vi "ProcessAlways.vi"(0 "StateIn":T2 {"ILoad" format="%_6g"; "Fault Registers" format="%016x"; "VLoad" format="%_6g"; "VDCLink" format="%_6g"; "Detected Frequency" format="%1_6g"}, 1 "Interfaces":T5, 11 "error in":errorcluster) -> (4 "StateOut":T2 {"ILoad" format="%_6g"; "Fault Registers" format="%016x"; "VLoad" format="%_6g"; "VDCLink" format="%_6g"; "Detected Frequency" format="%1_6g"}, 8 "method":T1, 10 "params":refnum<class "JSON Null.lvclass">, 15 "error out":errorcluster)   [LabVIEW 2017, in "AppStateMachine runtime.lvclass"]
uses:
  AppStateMachine runtime.lvclass
  Interfaces.ctl
  <vilib>/NI/NI JSONRPC Server Framework/Classes/Server/JSONRPC Server.lvclass
  <instrlib>/_niInstr/Instruction Framework/v1/Host/Instruction Target/niInstr Instruction Target v1 Host.lvclass
  <instrlib>/_niInstr/Instruction Framework/v1/Host/Instruction Framework Context/niInstr Instruction Framework Context v1 Host.lvclass
  FPGA/FPGAtypedef.ctl
  <vilib>/NI/PowerElectronicsControl/ThreePhasePLL/Interface/InterfaceRef.ctl
  <vilib>/NI/PowerElectronicsControl/ActiveFrontEnd/AFE_Interface/InterfaceRef.ctl
  <vilib>/NI/PowerElectronicsControl/Buck-Boost/RealTime/Interface.ctl
  State.ctl
  StateId.ctl
  LED_Color.ctl
  Support/methods.ctl
  <vilib>/NI/JSON Support for LabVIEW/JSON Data Classes/JSON Datatype/JSON Null.lvclass
  <vilib>/NI/NI JSONRPC Server Framework/Classes/Request/Request.lvclass/Request.ctl
  <vilib>/NI/NI JSONRPC Server Framework/Classes/Request/Read method.vi
  <vilib>/NI/NI JSONRPC Server Framework/Classes/Request/Read params.vi
  <vilib>/NI/JSON Support for LabVIEW/JSON Data Classes/JSON Object/JSON Object.lvclass
  C:/Program Files (x86)/National Instruments/LabVIEW 2017/vi.lib/NI/JSON Support for LabVIEW/JSON Data Classes/JSON Datatype/JSON Null.lvclass
  <vilib>/NI/JSON Support for LabVIEW/JSON Data Classes/JSON String/JSON String.lvclass
  <vilib>/NI/JSON Support for LabVIEW/JSON Data Classes/JSON Array/JSON Array.lvclass
  <vilib>/NI/NI JSONRPC Server Framework/Classes/Server/Add Response (Method Not Found from Request).vi
  <vilib>/NI/NI JSONRPC Server Framework/Classes/Server/Add Response (Result from Request).vi
  <vilib>/NI/JSON Support for LabVIEW/JSON Data Classes/JSON String/New JSON String.vi
  <vilib>/NI/JSON Support for LabVIEW/JSON Data Classes/JSON Array/New JSON Array (String).vi
  <vilib>/NI/JSON Support for LabVIEW/JSON Data Classes/JSON Array/New JSON Array (JSON Data).vi
  <vilib>/Utility/error.llb/Error Cluster From Error Code.vi
  <vilib>/rvi/errors/niLvFpgaAdjustHostInterfaceError.vi
  <vilib>/NI/JSON Support for LabVIEW/JSON Data Classes/JSON Object/New JSON Object (Empty).vi
  <vilib>/rvi/interface/nirviReadWriteControl/nirviReadWriteControl.xnode
  <vilib>/NI/NI JSONRPC Server Framework/Classes/params/params.lvclass
  <vilib>/rvi/interface/Simulation/niFpgaSimulationCallBeginRW.vi
  <vilib>/NI/PowerElectronicsControl/ThreePhasePLL/Interface/ThreePhasePLLInterface.lvlib
  <vilib>/NI/JSON Support for LabVIEW/JSON Data Classes/JSON Helper/JSON Helper.lvclass
  NiFpgaLv.dll
  <vilib>/NI/NI JSONRPC Server Framework/Classes/Request/Request.lvclass
  C:/Program Files (x86)/National Instruments/LabVIEW 2017/vi.lib/NI/JSON Support for LabVIEW/JSON Data Classes/JSON Basic Type/JSON Literal.lvclass
  C:/Program Files (x86)/National Instruments/LabVIEW 2017/vi.lib/NI/JSON Support for LabVIEW/JSON Data Classes/JSON Structured Type/JSON Structure.lvclass
  <vilib>/NI/PowerElectronicsControl/Buck-Boost/RealTime/BuckBoostInterface.lvlib
  <vilib>/NI/PowerElectronicsControl/ActiveFrontEnd/AFE_Interface/AFE_interface.lvlib
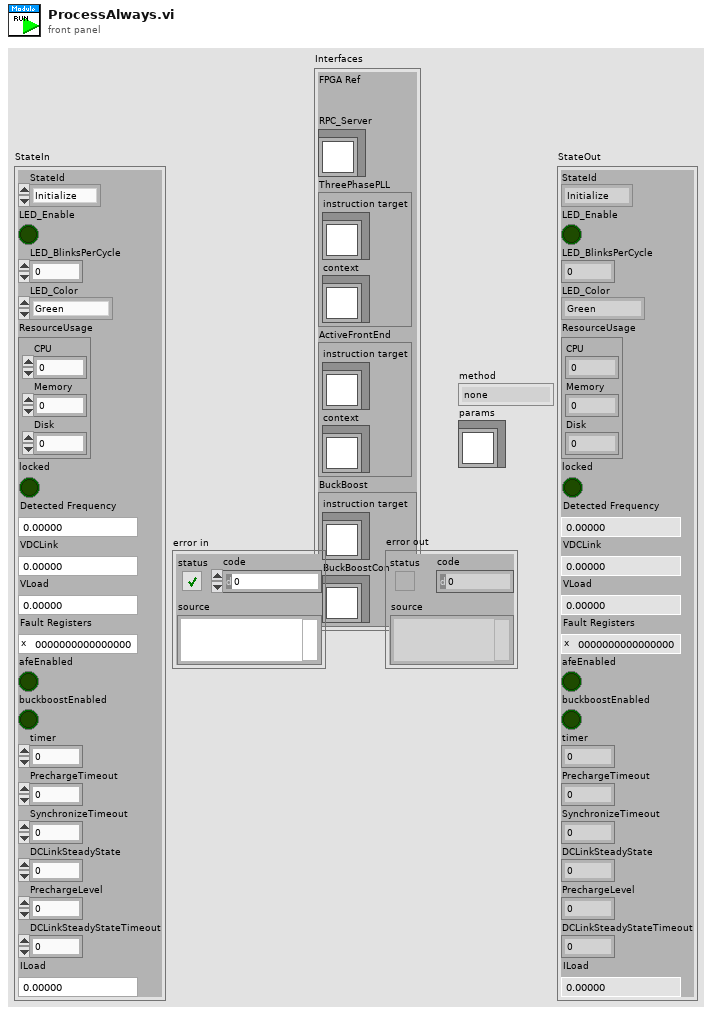
[diagram p1: front panel]
types:
  T1 = typedef "AppStateMachine runtime.lvclass/methods.ctl" = enum16{"none", "echo", "GetResourceUsage", "CheckConnection", "CurrentState", "GoToSafeState", "ClearSafeState", "AvailableLogs", "ForceLogTrigger", "GoToTuneAFE", "GoToTunePLL", "GoToTuneBuckBoost", "TurnOnSystem", "TurnOffSystem", "PrechargeSystem", "SetPLL_Tune", "SetBuckBoostSetpoint", "SetAFE_tune", "SetBuckBoostTune", "CompleteTuning", "PllSettings", "AfeSettings", "BuckBoostSettings", "enableAfe", "disableAfe", "enableBuckBoost", "disableBuckBoost"}
  T2 = typedef "AppStateMachine runtime.lvclass/State.ctl" = cluster{"StateId":T3, "LED_Enable":bool, "LED_BlinksPerCycle":i32, "LED_Color":T4, "ResourceUsage":cluster{"CPU":dbl, "Memory":dbl, "Disk":dbl}, "locked":bool, "Detected Frequency":dbl, "VDCLink":dbl, "VLoad":dbl, "Fault Registers":u64, "afeEnabled":bool, "buckboostEnabled":bool, "timer":u32, "PrechargeTimeout":u32, "SynchronizeTimeout":u32, "DCLinkSteadyState":dbl, "PrechargeLevel":dbl, "DCLinkSteadyStateTimeout":u32, "ILoad":dbl}
  T3 = typedef "AppStateMachine runtime.lvclass/StateId.ctl" = enum16{"Initialize", "Idle", "TunePLL", "TuneAFE", "TuneBuckBoost", "Precharge", "Synchronize", "Ready", "EnableAFE", "EnableBuckBoost", "Powered", "SafeState", "UnrecoverableSafeState"}
  T4 = typedef "AppStateMachine runtime.lvclass/LED_Color.ctl" = enum16{"Green", "Yellow"}
  T5 = typedef "AppStateMachine runtime.lvclass/Interfaces.ctl" = cluster{"FPGA Ref":T6, "RPC_Server":refnum<class "JSONRPC Server.lvclass">, "ThreePhasePLL":T7, "ActiveFrontEnd":T8, "BuckBoost":T9}
  T6 = typedef "AppStateMachine runtime.lvclass/FPGAtypedef.ctl" = refnum<k20>
  T7 = typedef "ThreePhasePLLInterface.lvlib/InterfaceRef.ctl" = cluster{"instruction target":refnum<class "niInstr Instruction Target v1 Host.lvclass">, "context":refnum<class "niInstr Instruction Framework Context v1 Host.lvclass">}
  T8 = typedef "AFE_interface.lvlib/InterfaceRef.ctl" = cluster{"instruction target":refnum<class "niInstr Instruction Target v1 Host.lvclass">, "context":refnum<class "niInstr Instruction Framework Context v1 Host.lvclass">}
  T9 = typedef "BuckBoostInterface.lvlib/Interface.ctl" = cluster{"instruction target":refnum<class "niInstr Instruction Target v1 Host.lvclass">, "BuckBoostContext":refnum<class "niInstr Instruction Framework Context v1 Host.lvclass">}
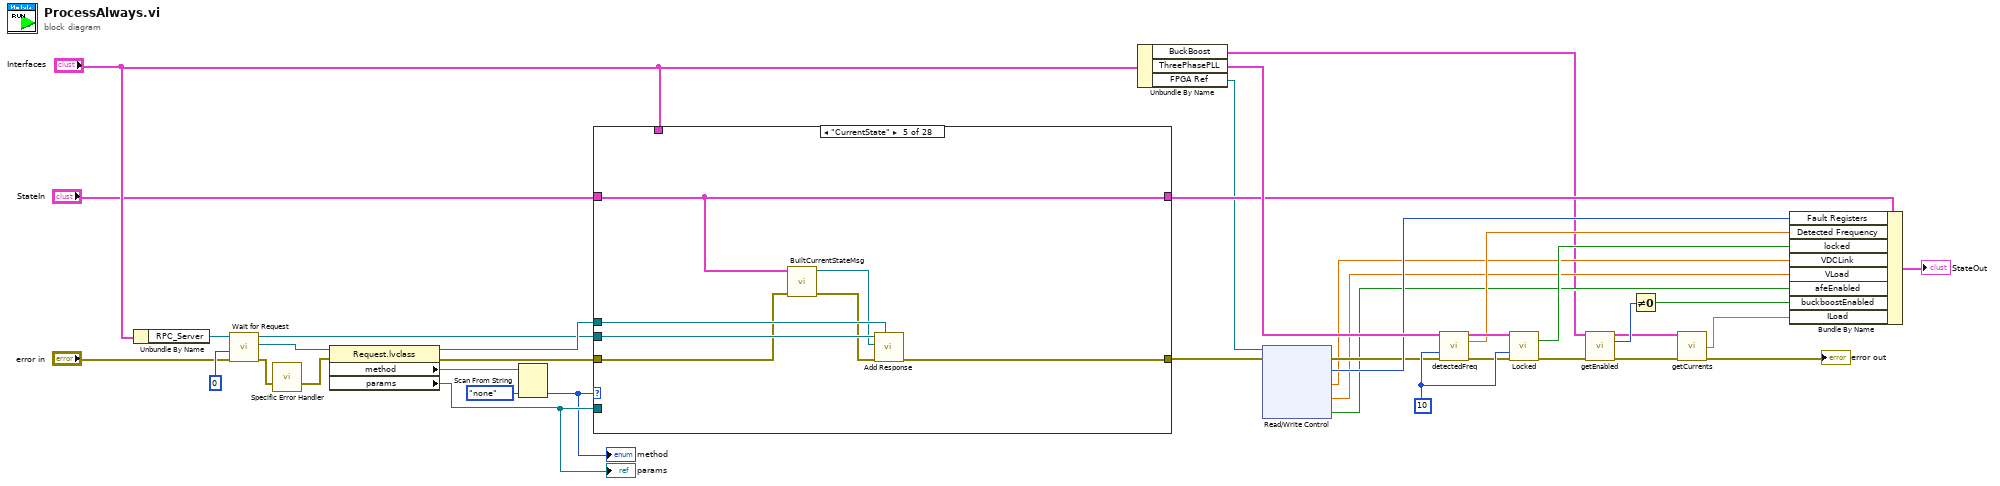
[diagram p0: block diagram]
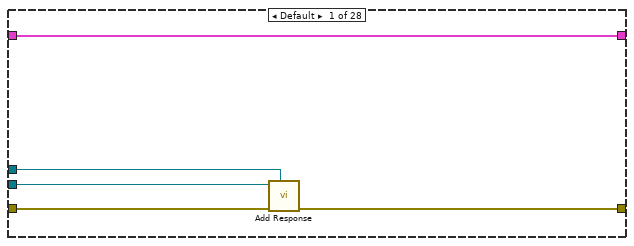
[diagram p2: hidden frame]
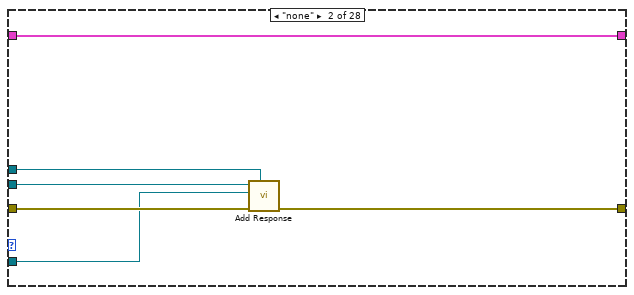
[diagram p3: hidden frame]
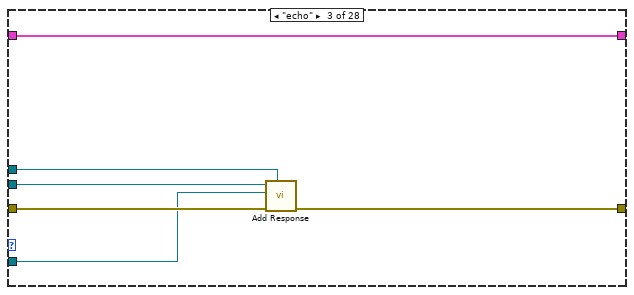
[diagram p4: hidden frame]
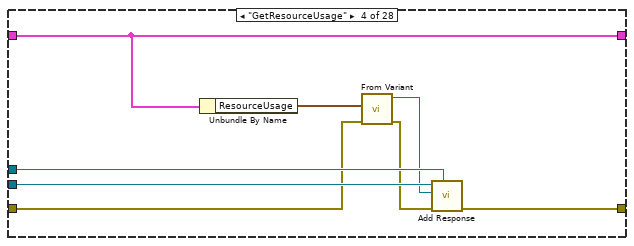
[diagram p5: hidden frame]
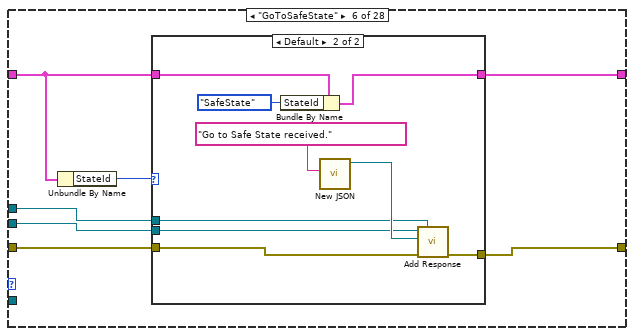
[diagram p6: hidden frame]
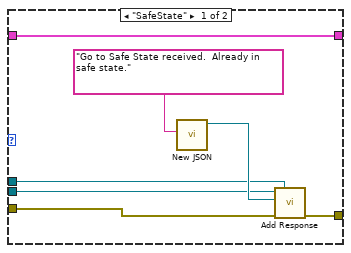
[diagram p7: hidden frame]
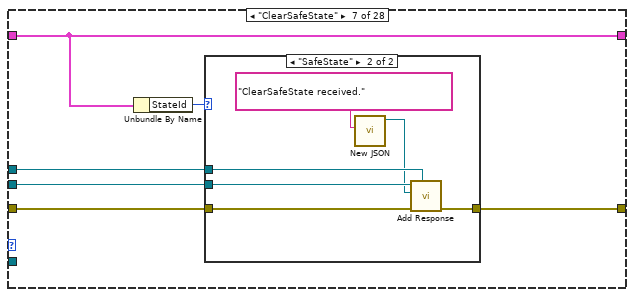
[diagram p8: hidden frame]
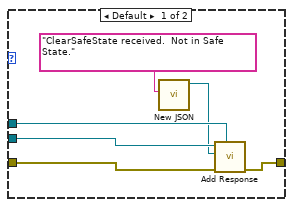
[diagram p9: hidden frame]
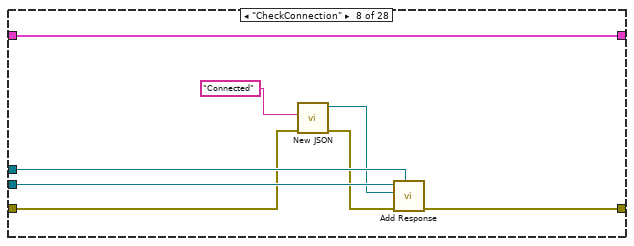
[diagram p10: hidden frame]
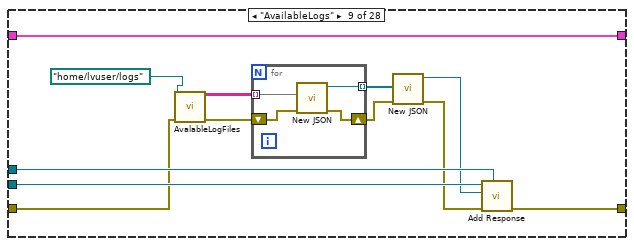
[diagram p11: hidden frame]
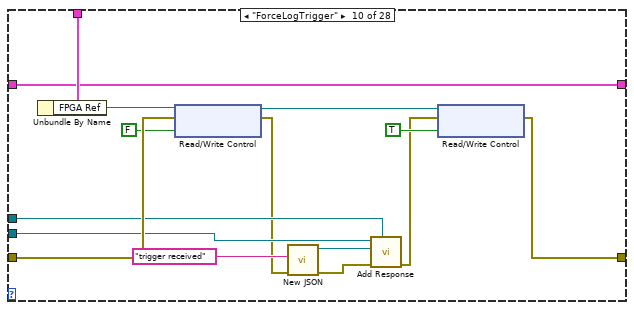
[diagram p12: hidden frame]
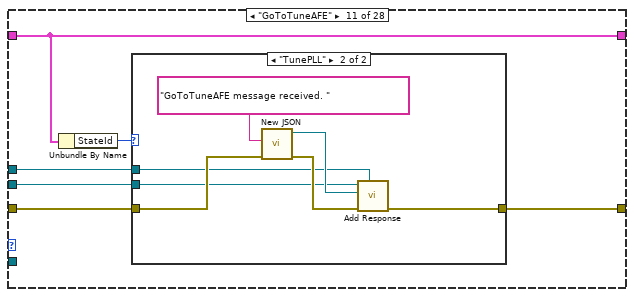
[diagram p13: hidden frame]
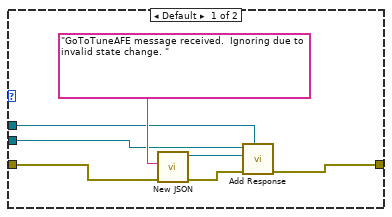
[diagram p14: hidden frame]
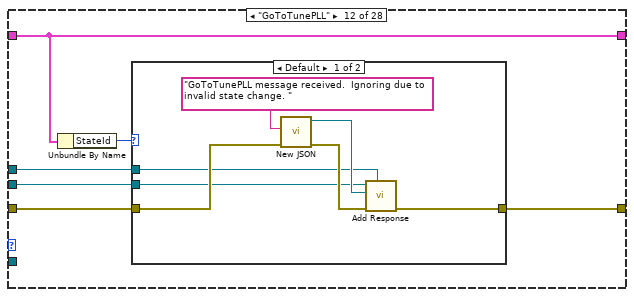
[diagram p15: hidden frame]
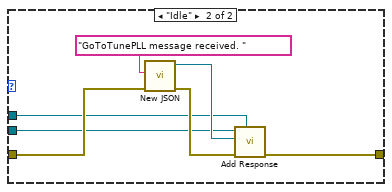
[diagram p16: hidden frame]
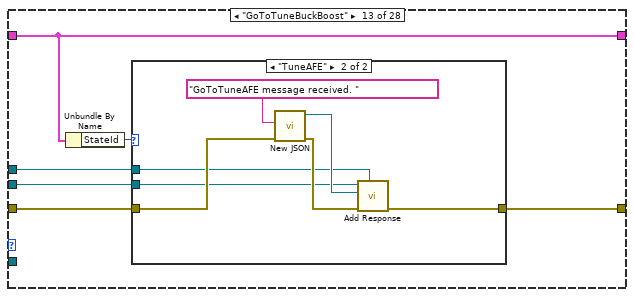
[diagram p17: hidden frame]
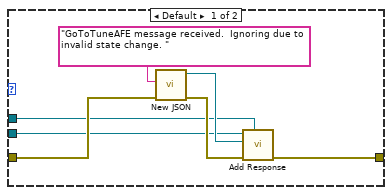
[diagram p18: hidden frame]
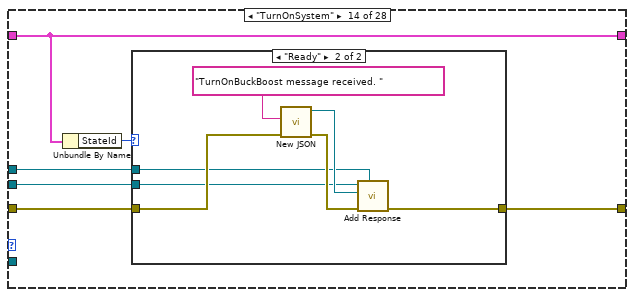
[diagram p19: hidden frame]
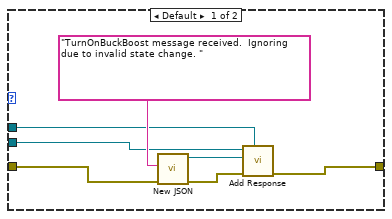
[diagram p20: hidden frame]
diagram:
  w34 = 10 ("timeout (5000 ms)")
  n1 = Unbundle By Name("Interfaces") -> ("RPC_Server"=w21:refnum<class "JSONRPC Server.lvclass">)
  n2 = call <vilib>:"Wait for Request.vi"("error in (no error)"="error in", "timeout in ms (100)"=0, "Server in"=w21) -> ("error out"=w29:errorcluster, "Request"=w28:refnum<class "Request.lvclass">, "Server out"=w22:refnum<class "JSONRPC Server.lvclass">)  [unwired: 5 in, 1 out]
  n3 = call "Specific Error Handler"("Error to Check"=w29) -> ("error out"=w27:errorcluster)  [unwired: 11 in, 3 out]
  n4 = property class="Request.lvclass"(reference=w28, error in=w27) -> (reference out=w23:refnum<class "Request.lvclass">, error out=w25:errorcluster, "method"=w24:string, "params"=w32:refnum<class "JSON Null.lvclass">)
  "params" <- w32
  n5 = Scan From String(input string=w24, default 1=methods."none" ("methods")) -> (output 1=w31:T1)  [unwired: 3 in, 3 out]
  "method" <- w31
  n6 = case shown="\"CurrentState\"" w31 {
    tunnel: w32 -> [_ w46 w51 _ _ _ _ _ _ _ _ _ _ _ _ _ _ _ _ _ _ _ _ _ _ _ _ _]
    tunnel: w25 -> [w41 w48 w53 w59 w66 w77 w98 w115 w128 w150 w156 w176 w196 w216 w236 w256 w276 w296 w316 w336 w356 w376 w396 w416 w436 w453 w473 w493]
    tunnel: w23 -> [w40 w47 w54 w62 w69 w74 w96 w118 w129 w149 w154 w174 w194 w214 w234 w254 w274 w294 w314 w334 w354 w374 w394 w414 w434 w457 w477 w497]
    tunnel: w22 -> [w42 w45 w55 w61 w68 w75 w95 w117 w130 w148 w153 w173 w193 w213 w233 w253 w273 w293 w313 w333 w353 w373 w393 w413 w433 w458 w478 w498]
    tunnel: [w39 w44 w52 w63 w70 w76 w97 w119 w131 w143 w155 w175 w195 w215 w235 w255 w275 w295 w315 w335 w355 w375 w395 w415 w435 w459 w479 w499] -> w15
    tunnel: "StateIn" -> [w43 w49 w50 w56 w67 w72 w94 w112 w120 w136 w151 w171 w192 w212 w231 w252 w271 w292 w312 w332 w352 w372 w391 w411 w432 w463 w483 w503]
    tunnel: "Interfaces" -> [_ _ _ _ _ _ _ _ _ w138 _ _ _ _ _ _ _ _ _ _ _ _ _ _ _ _ _ _]
    tunnel: [w43 w49 w50 w56 w67 w71 w94 w112 w120 w136 w151 w171 w192 w212 w231 w252 w271 w292 w312 w332 w352 w372 w391 w411 w432 w463 w483 w503] -> w17
    frame Default {
      n7 = call-poly <vilib>:"Add Response.vi"("Request"=w40, "error in (no error)"=w41, "Server in"=w42) -> ("error out"=w39:errorcluster)  [unwired: 6 in, 2 out]
    }
    frame "none" {
      n8 = call-poly <vilib>:"Add Response.vi"("Request"=w47, "error in (no error)"=w48, "JSON in"=w46, "Server in"=w45) -> ("error out"=w44:errorcluster)  [unwired: 5 in, 2 out]
    }
    frame "echo" {
      n9 = call-poly <vilib>:"Add Response.vi"("Request"=w54, "error in (no error)"=w53, "JSON in"=w51, "Server in"=w55) -> ("error out"=w52:errorcluster)  [unwired: 5 in, 2 out]
    }
    frame "GetResourceUsage" {
      n10 = Unbundle By Name(w56) -> ("ResourceUsage"=w57:cluster{"CPU":dbl, "Memory":dbl, "Disk":dbl})
      n11 = call <vilib>:"From Variant.vi"("error in (no error)"=w59, "Variant"=w57) -> ("error out"=w58:errorcluster, "JSON out"=w60:refnum<class "JSON Null.lvclass">)  [unwired: 8 in]
      n12 = call-poly <vilib>:"Add Response.vi"("Request"=w62, "error in (no error)"=w58, "JSON in"=w60, "Server in"=w61) -> ("error out"=w63:errorcluster)  [unwired: 5 in, 2 out]
    }
    frame "CurrentState" {
      n13 = call "BuiltCurrentStateMsg.vi"("State"=w67, "error in (no error)"=w66) -> ("CurrentStateMsg"=w64:refnum<class "JSON Object.lvclass">, "error out"=w65:errorcluster)  [unwired: 12 in]
      n14 = call-poly <vilib>:"Add Response.vi"("Request"=w69, "error in (no error)"=w65, "JSON in"=w64, "Server in"=w68) -> ("error out"=w70:errorcluster)  [unwired: 5 in, 2 out]
    }
    frame "GoToSafeState" {
      n15 = Unbundle By Name(w72) -> ("StateId"=w73:T3)
      n16 = case shown="Default" w73 {
        tunnel: w77 -> [w84 w93]
        tunnel: [w83 w92] -> w76
        tunnel: w75 -> [w80 w89]
        tunnel: w74 -> [w79 w88]
        tunnel: w72 -> [w78 w87]
        tunnel: [w78 w85] -> w71
        frame "SafeState" {
          n17 = call-poly <vilib>:"New JSON.vi"("value"="Go to Safe State received.  Already in safe state.") -> ("JSON String out"=w81:refnum<class "JSON String.lvclass">)  [unwired: 9 in, 1 out]
          n18 = call-poly <vilib>:"Add Response.vi"("Request"=w79, "error in (no error)"=w84, "JSON in"=w81, "Server in"=w80) -> ("error out"=w83:errorcluster)  [unwired: 5 in, 2 out]
        }
        frame Default {
          n19 = Bundle By Name(cluster=w87, "StateId"=StateId."SafeState") -> (w85:T2)
          n20 = call-poly <vilib>:"New JSON.vi"("value"="Go to Safe State received.") -> ("JSON String out"=w90:refnum<class "JSON String.lvclass">)  [unwired: 9 in, 1 out]
          n21 = call-poly <vilib>:"Add Response.vi"("Request"=w88, "error in (no error)"=w93, "JSON in"=w90, "Server in"=w89) -> ("error out"=w92:errorcluster)  [unwired: 5 in, 2 out]
        }
      }
    }
    frame "ClearSafeState" {
      n22 = Unbundle By Name(w94) -> ("StateId"=w99:T3)
      n23 = case shown="\"SafeState\"" w99 {
        tunnel: w98 -> [w104 w110]
        tunnel: [w105 w111] -> w97
        tunnel: w96 -> [w103 w109]
        tunnel: w95 -> [w102 w108]
        frame Default {
          n24 = call-poly <vilib>:"New JSON.vi"("value"="ClearSafeState received.  Not in Safe State." ("String")) -> ("JSON String out"=w100:refnum<class "JSON String.lvclass">)  [unwired: 9 in, 1 out]
          n25 = call-poly <vilib>:"Add Response.vi"("Request"=w103, "error in (no error)"=w104, "JSON in"=w100, "Server in"=w102) -> ("error out"=w105:errorcluster)  [unwired: 5 in, 2 out]
        }
        frame "SafeState" {
          n26 = call-poly <vilib>:"New JSON.vi"("value"="ClearSafeState received." ("String")) -> ("JSON String out"=w106:refnum<class "JSON String.lvclass">)  [unwired: 9 in, 1 out]
          n27 = call-poly <vilib>:"Add Response.vi"("Request"=w109, "error in (no error)"=w110, "JSON in"=w106, "Server in"=w108) -> ("error out"=w111:errorcluster)  [unwired: 5 in, 2 out]
        }
      }
    }
    frame "CheckConnection" {
      n28 = call-poly <vilib>:"New JSON.vi"("error in (no error)"=w115, "value"="Connected" ("String")) -> ("error out"=w113:errorcluster, "JSON String out"=w114:refnum<class "JSON String.lvclass">)  [unwired: 8 in]
      n29 = call-poly <vilib>:"Add Response.vi"("Request"=w118, "error in (no error)"=w113, "JSON in"=w114, "Server in"=w117) -> ("error out"=w119:errorcluster)  [unwired: 5 in, 2 out]
    }
    frame "AvailableLogs" {
      n30 = call "AvalableLogFiles.vi"("path"=path "/home/lvuser/logs", "error in (no error)"=w128) -> ("FilesInfo"=w126:string[][], "error out"=w125:errorcluster)  [unwired: 12 in]
      n31 = for {
        tunnel: w126 -> [w135] mode=indexing
        shift-right: [w133] -> w123
        shift-left: w125 -> [w134]
        tunnel: [w132] -> w124 mode=indexing
        n32 = call-poly <vilib>:"New JSON.vi"("error in (no error)"=w134, "String Array"=w135) -> ("error out"=w133:errorcluster, "JSON Array out"=w132:refnum<class "JSON Array.lvclass">)  [unwired: 8 in]
      }
      n33 = call-poly <vilib>:"New JSON.vi"("error in (no error)"=w123, "JSON Datatypes"=w124) -> ("error out"=w122:errorcluster, "JSON Array out"=w121:refnum<class "JSON Array.lvclass">)  [unwired: 8 in]
      n34 = call-poly <vilib>:"Add Response.vi"("Request"=w129, "error in (no error)"=w122, "JSON in"=w121, "Server in"=w130) -> ("error out"=w131:errorcluster)  [unwired: 5 in, 2 out]
    }
    frame "ForceLogTrigger" {
      n35 = Unbundle By Name(w138) -> ("FPGA Ref"=w137:T6)
      n36 = xnode "Read/Write Control"("FPGA VI Reference In"=w137, "error in"=w150, "ManualTrigger"=FALSE) -> ("FPGA VI Reference Out"=w146:T6, "error out"=w140:errorcluster)
      n37 = call-poly <vilib>:"New JSON.vi"("error in (no error)"=w140, "value"="trigger received" ("String")) -> ("error out"=w139:errorcluster, "JSON String out"=w142:refnum<class "JSON String.lvclass">)  [unwired: 8 in]
      n38 = call-poly <vilib>:"Add Response.vi"("Request"=w149, "error in (no error)"=w139, "JSON in"=w142, "Server in"=w148) -> ("error out"=w144:errorcluster)  [unwired: 5 in, 2 out]
      n39 = xnode "Read/Write Control"("FPGA VI Reference In"=w146, "error in"=w144, "ManualTrigger"=TRUE) -> ("error out"=w143:errorcluster)  [unwired: 1 out]
    }
    frame "GoToTuneAFE" {
      n40 = Unbundle By Name(w151) -> ("StateId"=w152:T3)
      n41 = case shown="\"TunePLL\"" w152 {
        tunnel: w156 -> [w160 w168]
        tunnel: [w159 w166] -> w155
        tunnel: w154 -> [w158 w164]
        tunnel: w153 -> [w157 w165]
        frame Default {
          n42 = call-poly <vilib>:"New JSON.vi"("error in (no error)"=w160, "value"="GoToTuneAFE message received.  Ignoring due to invalid state change. " ("String")) -> ("error out"=w161:errorcluster, "JSON String out"=w163:refnum<class "JSON String.lvclass">)  [unwired: 8 in]
          n43 = call-poly <vilib>:"Add Response.vi"("Request"=w158, "error in (no error)"=w161, "JSON in"=w163, "Server in"=w157) -> ("error out"=w159:errorcluster)  [unwired: 5 in, 2 out]
        }
        frame "TunePLL" {
          n44 = call-poly <vilib>:"New JSON.vi"("error in (no error)"=w168, "value"="GoToTuneAFE message received. " ("String")) -> ("error out"=w167:errorcluster, "JSON String out"=w170:refnum<class "JSON String.lvclass">)  [unwired: 8 in]
          n45 = call-poly <vilib>:"Add Response.vi"("Request"=w164, "error in (no error)"=w167, "JSON in"=w170, "Server in"=w165) -> ("error out"=w166:errorcluster)  [unwired: 5 in, 2 out]
        }
      }
    }
    frame "GoToTunePLL" {
      n46 = Unbundle By Name(w171) -> ("StateId"=w172:T3)
      n47 = case shown="Default" w172 {
        tunnel: w176 -> [w180 w188]
        tunnel: [w179 w186] -> w175
        tunnel: w174 -> [w178 w185]
        tunnel: w173 -> [w177 w184]
        frame Default {
          n48 = call-poly <vilib>:"New JSON.vi"("error in (no error)"=w180, "value"="GoToTunePLL message received.  Ignoring due to invalid state change. " ("String")) -> ("error out"=w181:errorcluster, "JSON String out"=w183:refnum<class "JSON String.lvclass">)  [unwired: 8 in]
          n49 = call-poly <vilib>:"Add Response.vi"("Request"=w178, "error in (no error)"=w181, "JSON in"=w183, "Server in"=w177) -> ("error out"=w179:errorcluster)  [unwired: 5 in, 2 out]
        }
        frame "Idle" {
          n50 = call-poly <vilib>:"New JSON.vi"("error in (no error)"=w188, "value"="GoToTunePLL message received. " ("String")) -> ("error out"=w187:errorcluster, "JSON String out"=w190:refnum<class "JSON String.lvclass">)  [unwired: 8 in]
          n51 = call-poly <vilib>:"Add Response.vi"("Request"=w185, "error in (no error)"=w187, "JSON in"=w190, "Server in"=w184) -> ("error out"=w186:errorcluster)  [unwired: 5 in, 2 out]
        }
      }
    }
    frame "GoToTuneBuckBoost" {
      n52 = Unbundle By Name(w192) -> ("StateId"=w191:T3)
      n53 = case shown="\"TuneAFE\"" w191 {
        tunnel: w196 -> [w200 w208]
        tunnel: [w199 w206] -> w195
        tunnel: w194 -> [w198 w205]
        tunnel: w193 -> [w197 w204]
        frame Default {
          n54 = call-poly <vilib>:"New JSON.vi"("error in (no error)"=w200, "value"="GoToTuneAFE message received.  Ignoring due to invalid state change. " ("String")) -> ("error out"=w201:errorcluster, "JSON String out"=w203:refnum<class "JSON String.lvclass">)  [unwired: 8 in]
          n55 = call-poly <vilib>:"Add Response.vi"("Request"=w198, "error in (no error)"=w201, "JSON in"=w203, "Server in"=w197) -> ("error out"=w199:errorcluster)  [unwired: 5 in, 2 out]
        }
        frame "TuneAFE" {
          n56 = call-poly <vilib>:"New JSON.vi"("error in (no error)"=w208, "value"="GoToTuneAFE message received. " ("String")) -> ("error out"=w207:errorcluster, "JSON String out"=w210:refnum<class "JSON String.lvclass">)  [unwired: 8 in]
          n57 = call-poly <vilib>:"Add Response.vi"("Request"=w205, "error in (no error)"=w207, "JSON in"=w210, "Server in"=w204) -> ("error out"=w206:errorcluster)  [unwired: 5 in, 2 out]
        }
      }
    }
    frame "TurnOnSystem" {
      n58 = Unbundle By Name(w212) -> ("StateId"=w211:T3)
      n59 = case shown="\"Ready\"" w211 {
        tunnel: w216 -> [w220 w228]
        tunnel: [w219 w226] -> w215
        tunnel: w214 -> [w218 w225]
        tunnel: w213 -> [w217 w224]
        frame Default {
          n60 = call-poly <vilib>:"New JSON.vi"("error in (no error)"=w220, "value"="TurnOnBuckBoost message received.  Ignoring due to invalid state change. " ("String")) -> ("error out"=w221:errorcluster, "JSON String out"=w223:refnum<class "JSON String.lvclass">)  [unwired: 8 in]
          n61 = call-poly <vilib>:"Add Response.vi"("Request"=w218, "error in (no error)"=w221, "JSON in"=w223, "Server in"=w217) -> ("error out"=w219:errorcluster)  [unwired: 5 in, 2 out]
        }
        frame "Ready" {
          n62 = call-poly <vilib>:"New JSON.vi"("error in (no error)"=w228, "value"="TurnOnBuckBoost message received. " ("String")) -> ("error out"=w227:errorcluster, "JSON String out"=w230:refnum<class "JSON String.lvclass">)  [unwired: 8 in]
          n63 = call-poly <vilib>:"Add Response.vi"("Request"=w225, "error in (no error)"=w227, "JSON in"=w230, "Server in"=w224) -> ("error out"=w226:errorcluster)  [unwired: 5 in, 2 out]
        }
      }
    }
    frame "TurnOffSystem" {
      n64 = Unbundle By Name(w231) -> ("StateId"=w232:T3)
      n65 = case shown="\"Ready\", \"Powered\"" w232 {
        tunnel: w236 -> [w240 w248]
        tunnel: [w239 w246] -> w235
        tunnel: w234 -> [w238 w245]
        tunnel: w233 -> [w237 w244]
        frame Default {
          n66 = call-poly <vilib>:"New JSON.vi"("error in (no error)"=w240, "value"="TurnOffSystem message received.  Ignoring due to invalid state change. " ("String")) -> ("error out"=w241:errorcluster, "JSON String out"=w243:refnum<class "JSON String.lvclass">)  [unwired: 8 in]
          n67 = call-poly <vilib>:"Add Response.vi"("Request"=w238, "error in (no error)"=w241, "JSON in"=w243, "Server in"=w237) -> ("error out"=w239:errorcluster)  [unwired: 5 in, 2 out]
        }
        frame "Ready", "Powered" {
          n68 = call-poly <vilib>:"New JSON.vi"("error in (no error)"=w248, "value"="TurnOffSystem message received. " ("String")) -> ("error out"=w247:errorcluster, "JSON String out"=w250:refnum<class "JSON String.lvclass">)  [unwired: 8 in]
          n69 = call-poly <vilib>:"Add Response.vi"("Request"=w245, "error in (no error)"=w247, "JSON in"=w250, "Server in"=w244) -> ("error out"=w246:errorcluster)  [unwired: 5 in, 2 out]
        }
      }
    }
    frame "PrechargeSystem" {
      n70 = Unbundle By Name(w252) -> ("StateId"=w251:T3)
      n71 = case shown="Default" w251 {
        tunnel: w256 -> [w260 w268]
        tunnel: [w259 w266] -> w255
        tunnel: w254 -> [w258 w265]
        tunnel: w253 -> [w257 w264]
        frame Default {
          n72 = call-poly <vilib>:"New JSON.vi"("error in (no error)"=w260, "value"="PrechargeSystem message received.  Ignoring due to invalid state change. " ("String")) -> ("error out"=w261:errorcluster, "JSON String out"=w263:refnum<class "JSON String.lvclass">)  [unwired: 8 in]
          n73 = call-poly <vilib>:"Add Response.vi"("Request"=w258, "error in (no error)"=w261, "JSON in"=w263, "Server in"=w257) -> ("error out"=w259:errorcluster)  [unwired: 5 in, 2 out]
        }
        frame "Idle" {
          n74 = call-poly <vilib>:"New JSON.vi"("error in (no error)"=w268, "value"="PrechargeSystem message received. " ("String")) -> ("error out"=w267:errorcluster, "JSON String out"=w270:refnum<class "JSON String.lvclass">)  [unwired: 8 in]
          n75 = call-poly <vilib>:"Add Response.vi"("Request"=w265, "error in (no error)"=w267, "JSON in"=w270, "Server in"=w264) -> ("error out"=w266:errorcluster)  [unwired: 5 in, 2 out]
        }
      }
    }
    frame "SetPLL_Tune" {
      n76 = Unbundle By Name(w271) -> ("StateId"=w272:T3)
      n77 = case shown="\"TunePLL\"" w272 {
        tunnel: w276 -> [w280 w288]
        tunnel: [w279 w286] -> w275
        tunnel: w274 -> [w278 w285]
        tunnel: w273 -> [w277 w284]
        frame Default {
          n78 = call-poly <vilib>:"New JSON.vi"("error in (no error)"=w280, "value"="SetPLL_Tune message received.  Ignoring because not in TunePLL State. " ("String")) -> ("error out"=w281:errorcluster, "JSON String out"=w283:refnum<class "JSON String.lvclass">)  [unwired: 8 in]
          n79 = call-poly <vilib>:"Add Response.vi"("Request"=w278, "error in (no error)"=w281, "JSON in"=w283, "Server in"=w277) -> ("error out"=w279:errorcluster)  [unwired: 5 in, 2 out]
        }
        frame "TunePLL" {
          n80 = call-poly <vilib>:"New JSON.vi"("error in (no error)"=w288, "value"="SetPLL_Tune message received. " ("String")) -> ("error out"=w287:errorcluster, "JSON String out"=w290:refnum<class "JSON String.lvclass">)  [unwired: 8 in]
          n81 = call-poly <vilib>:"Add Response.vi"("Request"=w285, "error in (no error)"=w287, "JSON in"=w290, "Server in"=w284) -> ("error out"=w286:errorcluster)  [unwired: 5 in, 2 out]
        }
      }
    }
    frame "SetBuckBoostSetpoint" {
      n82 = Unbundle By Name(w292) -> ("StateId"=w291:T3)
      n83 = case shown="Default" w291 {
        tunnel: w296 -> [w300 w308]
        tunnel: [w299 w306] -> w295
        tunnel: w294 -> [w298 w305]
        tunnel: w293 -> [w297 w304]
        frame Default {
          n84 = call-poly <vilib>:"New JSON.vi"("error in (no error)"=w300, "value"="SetBuckBoostSetpoint message received.  Ignoring because not in Powered State. " ("String")) -> ("error out"=w301:errorcluster, "JSON String out"=w303:refnum<class "JSON String.lvclass">)  [unwired: 8 in]
          n85 = call-poly <vilib>:"Add Response.vi"("Request"=w298, "error in (no error)"=w301, "JSON in"=w303, "Server in"=w297) -> ("error out"=w299:errorcluster)  [unwired: 5 in, 2 out]
        }
        frame "Powered" {
          n86 = call-poly <vilib>:"New JSON.vi"("error in (no error)"=w308, "value"="SetBuckBoostValue message received. " ("String")) -> ("error out"=w307:errorcluster, "JSON String out"=w310:refnum<class "JSON String.lvclass">)  [unwired: 8 in]
          n87 = call-poly <vilib>:"Add Response.vi"("Request"=w305, "error in (no error)"=w307, "JSON in"=w310, "Server in"=w304) -> ("error out"=w306:errorcluster)  [unwired: 5 in, 2 out]
        }
      }
    }
    frame "enableAfe" {
      n88 = Unbundle By Name(w312) -> ("StateId"=w311:T3)
      n89 = case shown="\"TuneAFE\"" w311 {
        tunnel: w316 -> [w320 w328]
        tunnel: [w319 w326] -> w315
        tunnel: w314 -> [w318 w325]
        tunnel: w313 -> [w317 w324]
        frame Default {
          n90 = call-poly <vilib>:"New JSON.vi"("error in (no error)"=w320, "value"="enableAfe message received.  Ignoring because not in TuneAFE state. " ("String")) -> ("error out"=w321:errorcluster, "JSON String out"=w323:refnum<class "JSON String.lvclass">)  [unwired: 8 in]
          n91 = call-poly <vilib>:"Add Response.vi"("Request"=w318, "error in (no error)"=w321, "JSON in"=w323, "Server in"=w317) -> ("error out"=w319:errorcluster)  [unwired: 5 in, 2 out]
        }
        frame "TuneAFE" {
          n92 = call-poly <vilib>:"New JSON.vi"("error in (no error)"=w328, "value"="enableAfe message received. " ("String")) -> ("error out"=w327:errorcluster, "JSON String out"=w330:refnum<class "JSON String.lvclass">)  [unwired: 8 in]
          n93 = call-poly <vilib>:"Add Response.vi"("Request"=w325, "error in (no error)"=w327, "JSON in"=w330, "Server in"=w324) -> ("error out"=w326:errorcluster)  [unwired: 5 in, 2 out]
        }
      }
    }
    frame "disableAfe" {
      n94 = Unbundle By Name(w332) -> ("StateId"=w331:T3)
      n95 = case shown="\"TuneAFE\"" w331 {
        tunnel: w336 -> [w340 w348]
        tunnel: [w339 w346] -> w335
        tunnel: w334 -> [w338 w345]
        tunnel: w333 -> [w337 w344]
        frame Default {
          n96 = call-poly <vilib>:"New JSON.vi"("error in (no error)"=w340, "value"="disableAfe message received.  Ignoring because not in TuneAFE state. " ("String")) -> ("error out"=w341:errorcluster, "JSON String out"=w343:refnum<class "JSON String.lvclass">)  [unwired: 8 in]
          n97 = call-poly <vilib>:"Add Response.vi"("Request"=w338, "error in (no error)"=w341, "JSON in"=w343, "Server in"=w337) -> ("error out"=w339:errorcluster)  [unwired: 5 in, 2 out]
        }
        frame "TuneAFE" {
          n98 = call-poly <vilib>:"New JSON.vi"("error in (no error)"=w348, "value"="disableAfe message received. " ("String")) -> ("error out"=w347:errorcluster, "JSON String out"=w350:refnum<class "JSON String.lvclass">)  [unwired: 8 in]
          n99 = call-poly <vilib>:"Add Response.vi"("Request"=w345, "error in (no error)"=w347, "JSON in"=w350, "Server in"=w344) -> ("error out"=w346:errorcluster)  [unwired: 5 in, 2 out]
        }
      }
    }
    frame "enableBuckBoost" {
      n100 = Unbundle By Name(w352) -> ("StateId"=w351:T3)
      n101 = case shown="\"TuneBuckBoost\"" w351 {
        tunnel: w356 -> [w360 w368]
        tunnel: [w359 w366] -> w355
        tunnel: w354 -> [w358 w365]
        tunnel: w353 -> [w357 w364]
        frame Default {
          n102 = call-poly <vilib>:"New JSON.vi"("error in (no error)"=w360, "value"="enableBuckBoost message received.  Ignoring because not in TuneBuckBoost state. " ("String")) -> ("error out"=w361:errorcluster, "JSON String out"=w363:refnum<class "JSON String.lvclass">)  [unwired: 8 in]
          n103 = call-poly <vilib>:"Add Response.vi"("Request"=w358, "error in (no error)"=w361, "JSON in"=w363, "Server in"=w357) -> ("error out"=w359:errorcluster)  [unwired: 5 in, 2 out]
        }
        frame "TuneBuckBoost" {
          n104 = call-poly <vilib>:"New JSON.vi"("error in (no error)"=w368, "value"="enableBuckBoost message received. " ("String")) -> ("error out"=w367:errorcluster, "JSON String out"=w370:refnum<class "JSON String.lvclass">)  [unwired: 8 in]
          n105 = call-poly <vilib>:"Add Response.vi"("Request"=w365, "error in (no error)"=w367, "JSON in"=w370, "Server in"=w364) -> ("error out"=w366:errorcluster)  [unwired: 5 in, 2 out]
        }
      }
    }
    frame "disableBuckBoost" {
      n106 = Unbundle By Name(w372) -> ("StateId"=w371:T3)
      n107 = case shown="\"TuneBuckBoost\"" w371 {
        tunnel: w376 -> [w380 w388]
        tunnel: [w379 w386] -> w375
        tunnel: w374 -> [w378 w385]
        tunnel: w373 -> [w377 w384]
        frame Default {
          n108 = call-poly <vilib>:"New JSON.vi"("error in (no error)"=w380, "value"="disableBuckBoost message received.  Ignoring because not in TuneBuckBoost state. " ("String")) -> ("error out"=w381:errorcluster, "JSON String out"=w383:refnum<class "JSON String.lvclass">)  [unwired: 8 in]
          n109 = call-poly <vilib>:"Add Response.vi"("Request"=w378, "error in (no error)"=w381, "JSON in"=w383, "Server in"=w377) -> ("error out"=w379:errorcluster)  [unwired: 5 in, 2 out]
        }
        frame "TuneBuckBoost" {
          n110 = call-poly <vilib>:"New JSON.vi"("error in (no error)"=w388, "value"="disableBuckBoost message received. " ("String")) -> ("error out"=w387:errorcluster, "JSON String out"=w390:refnum<class "JSON String.lvclass">)  [unwired: 8 in]
          n111 = call-poly <vilib>:"Add Response.vi"("Request"=w385, "error in (no error)"=w387, "JSON in"=w390, "Server in"=w384) -> ("error out"=w386:errorcluster)  [unwired: 5 in, 2 out]
        }
      }
    }
    frame "SetAFE_tune" {
      n112 = Unbundle By Name(w391) -> ("StateId"=w392:T3)
      n113 = case shown="\"TuneAFE\"" w392 {
        tunnel: w396 -> [w400 w408]
        tunnel: [w399 w406] -> w395
        tunnel: w394 -> [w398 w405]
        tunnel: w393 -> [w397 w404]
        frame Default {
          n114 = call-poly <vilib>:"New JSON.vi"("error in (no error)"=w400, "value"="SetAFE_tune message received.  Ignoring because not in TuneAFE State. " ("String")) -> ("error out"=w401:errorcluster, "JSON String out"=w403:refnum<class "JSON String.lvclass">)  [unwired: 8 in]
          n115 = call-poly <vilib>:"Add Response.vi"("Request"=w398, "error in (no error)"=w401, "JSON in"=w403, "Server in"=w397) -> ("error out"=w399:errorcluster)  [unwired: 5 in, 2 out]
        }
        frame "TuneAFE" {
          n116 = call-poly <vilib>:"New JSON.vi"("error in (no error)"=w408, "value"="SetAFE_tune message received. " ("String")) -> ("error out"=w407:errorcluster, "JSON String out"=w410:refnum<class "JSON String.lvclass">)  [unwired: 8 in]
          n117 = call-poly <vilib>:"Add Response.vi"("Request"=w405, "error in (no error)"=w407, "JSON in"=w410, "Server in"=w404) -> ("error out"=w406:errorcluster)  [unwired: 5 in, 2 out]
        }
      }
    }
    frame "SetBuckBoostTune" {
      n118 = Unbundle By Name(w411) -> ("StateId"=w412:T3)
      n119 = case shown="Default" w412 {
        tunnel: w416 -> [w420 w428]
        tunnel: [w419 w426] -> w415
        tunnel: w414 -> [w418 w425]
        tunnel: w413 -> [w417 w424]
        frame Default {
          n120 = call-poly <vilib>:"New JSON.vi"("error in (no error)"=w420, "value"="SetBuckBoostTune message received.  Ignoring because not in TuneAFE State. " ("String")) -> ("error out"=w421:errorcluster, "JSON String out"=w423:refnum<class "JSON String.lvclass">)  [unwired: 8 in]
          n121 = call-poly <vilib>:"Add Response.vi"("Request"=w418, "error in (no error)"=w421, "JSON in"=w423, "Server in"=w417) -> ("error out"=w419:errorcluster)  [unwired: 5 in, 2 out]
        }
        frame "TuneBuckBoost" {
          n122 = call-poly <vilib>:"New JSON.vi"("error in (no error)"=w428, "value"="SetBuckBoostTune message received. " ("String")) -> ("error out"=w427:errorcluster, "JSON String out"=w430:refnum<class "JSON String.lvclass">)  [unwired: 8 in]
          n123 = call-poly <vilib>:"Add Response.vi"("Request"=w425, "error in (no error)"=w427, "JSON in"=w430, "Server in"=w424) -> ("error out"=w426:errorcluster)  [unwired: 5 in, 2 out]
        }
      }
    }
    frame "CompleteTuning" {
      n124 = Unbundle By Name(w432) -> ("StateId"=w431:T3)
      n125 = case shown="Default" w431 {
        tunnel: w436 -> [w440 w448]
        tunnel: [w439 w446] -> w435
        tunnel: w434 -> [w438 w445]
        tunnel: w433 -> [w437 w444]
        frame Default {
          n126 = call-poly <vilib>:"New JSON.vi"("error in (no error)"=w440, "value"="CompleteTuning message received.  Ignoring because not in TuneBuckBoost State. " ("String")) -> ("error out"=w441:errorcluster, "JSON String out"=w443:refnum<class "JSON String.lvclass">)  [unwired: 8 in]
          n127 = call-poly <vilib>:"Add Response.vi"("Request"=w438, "error in (no error)"=w441, "JSON in"=w443, "Server in"=w437) -> ("error out"=w439:errorcluster)  [unwired: 5 in, 2 out]
        }
        frame "TuneBuckBoost" {
          n128 = call-poly <vilib>:"New JSON.vi"("error in (no error)"=w448, "value"="CompleteTuning message received. " ("String")) -> ("error out"=w447:errorcluster, "JSON String out"=w450:refnum<class "JSON String.lvclass">)  [unwired: 8 in]
          n129 = call-poly <vilib>:"Add Response.vi"("Request"=w445, "error in (no error)"=w447, "JSON in"=w450, "Server in"=w444) -> ("error out"=w446:errorcluster)  [unwired: 5 in, 2 out]
        }
      }
    }
    frame "PllSettings" {
      n130 = Temporary Directory() -> (w462:path)
      n131 = Build Path(base path=w462, name or relative path="PllSettings.json") -> (appended path=w455:path)
      n132 = call <vilib>:"Check if File or Folder Exists.vi"("error in (no error)"=w453, "path"=w455) -> ("error out"=w454:errorcluster, "file or folder exists?"=w451:bool, "dup path"=w452:path)  [unwired: 7 in]
      n133 = case shown="True" w451 {
        tunnel: [w465 w470] -> w460
        tunnel: [w464 w469] -> w456
        tunnel: w454 -> [w466 w468]
        tunnel: w452 -> [_ w467]
        frame False {
          n134 = call-poly <vilib>:"New JSON.vi"("error in (no error)"=w466) -> ("error out"=w465:errorcluster, "JSON Object out"=w464:refnum<class "JSON Object.lvclass">)  [unwired: 9 in]
        }
        frame True {
          n135 = call <vilib>:"From File.vi"("error in"=w468, "file path"=w467) -> ("error out"=w470:errorcluster, "JSON out"=w469:refnum<class "JSON Null.lvclass">)  [unwired: 8 in]
        }
      }
      n136 = call-poly <vilib>:"Add Response.vi"("Request"=w457, "error in (no error)"=w460, "JSON in"=w456, "Server in"=w458) -> ("error out"=w459:errorcluster)  [unwired: 5 in, 2 out]
    }
    frame "AfeSettings" {
      n137 = Temporary Directory() -> (w482:path)
      n138 = Build Path(base path=w482, name or relative path="AfeSettings.json") -> (appended path=w475:path)
      n139 = call <vilib>:"Check if File or Folder Exists.vi"("error in (no error)"=w473, "path"=w475) -> ("error out"=w474:errorcluster, "file or folder exists?"=w471:bool, "dup path"=w472:path)  [unwired: 7 in]
      n140 = case shown="False" w471 {
        tunnel: [w485 w490] -> w480
        tunnel: [w484 w489] -> w476
        tunnel: w474 -> [w486 w488]
        tunnel: w472 -> [_ w487]
        frame False {
          n141 = call-poly <vilib>:"New JSON.vi"("error in (no error)"=w486) -> ("error out"=w485:errorcluster, "JSON Object out"=w484:refnum<class "JSON Object.lvclass">)  [unwired: 9 in]
        }
        frame True {
          n142 = call <vilib>:"From File.vi"("error in"=w488, "file path"=w487) -> ("error out"=w490:errorcluster, "JSON out"=w489:refnum<class "JSON Null.lvclass">)  [unwired: 8 in]
        }
      }
      n143 = call-poly <vilib>:"Add Response.vi"("Request"=w477, "error in (no error)"=w480, "JSON in"=w476, "Server in"=w478) -> ("error out"=w479:errorcluster)  [unwired: 5 in, 2 out]
    }
    frame "BuckBoostSettings" {
      n144 = Temporary Directory() -> (w502:path)
      n145 = Build Path(base path=w502, name or relative path="BuckBoostSettings.json") -> (appended path=w495:path)
      n146 = call <vilib>:"Check if File or Folder Exists.vi"("error in (no error)"=w493, "path"=w495) -> ("error out"=w494:errorcluster, "file or folder exists?"=w491:bool, "dup path"=w492:path)  [unwired: 7 in]
      n147 = case shown="False" w491 {
        tunnel: [w505 w510] -> w500
        tunnel: [w504 w509] -> w496
        tunnel: w494 -> [w506 w508]
        tunnel: w492 -> [_ w507]
        frame False {
          n148 = call-poly <vilib>:"New JSON.vi"("error in (no error)"=w506) -> ("error out"=w505:errorcluster, "JSON Object out"=w504:refnum<class "JSON Object.lvclass">)  [unwired: 9 in]
        }
        frame True {
          n149 = call <vilib>:"From File.vi"("error in"=w508, "file path"=w507) -> ("error out"=w510:errorcluster, "JSON out"=w509:refnum<class "JSON Null.lvclass">)  [unwired: 8 in]
        }
      }
      n150 = call-poly <vilib>:"Add Response.vi"("Request"=w497, "error in (no error)"=w500, "JSON in"=w496, "Server in"=w498) -> ("error out"=w499:errorcluster)  [unwired: 5 in, 2 out]
    }
  }
  n151 = Unbundle By Name("Interfaces") -> ("BuckBoost"=w7:T9, "ThreePhasePLL"=w37:T7, "FPGA Ref"=w14:T6)
  n152 = xnode "Read/Write Control"("FPGA VI Reference In"=w14, "error in"=w15) -> ("error out"=w16:errorcluster, "FaultBuffer"=w36:u64, "VDCLink"=w11:sgl, "VLoad"=w10:sgl, "enableAFE"=w9:bool)  [unwired: 1 out]
  n153 = call <vilib>:"detectedFreq.vi"("Interface in"=w37, "timeout (5000 ms)"=w34, "error in"=w16) -> ("Interface out"=w35:T7, "detectedFreq"=w12:sgl, "error out"=w33:errorcluster)  [unwired: 10 in]
  n154 = call <vilib>:"Locked.vi"("Interface in"=w35, "timeout (5000 ms)"=w34, "error in"=w33) -> ("Locked"=w13:bool, "error out"=w8:errorcluster)  [unwired: 10 in, 1 out]
  n155 = call <vilib>:"getEnabled.vi"("Interface in"=w7, "error in (no error)"=w8) -> ("Interface out"=w4:T9, "Enabled"=w6:u8, "error out"=w3:errorcluster)  [unwired: 11 in]
  n156 = Not Equal To 0?(x=w6) -> (x != 0?=w5:bool)
  n157 = call <vilib>:"getCurrents.vi"("Interface in"=w4, "error in (no error)"=w3) -> ("TotalCurrent"=w1:sgl, "error out"=→"error out":errorcluster)  [unwired: 10 in, 2 out]
  n158 = Bundle By Name(cluster=w17, "Fault Registers"=w36, "Detected Frequency"=w12, "locked"=w13, "VDCLink"=w11, "VLoad"=w10, "afeEnabled"=w9, "buckboostEnabled"=w5, "ILoad"=w1) -> (→"StateOut":T2)
